vi "Write Center Point.vi"(10 "Center Point":dbl[unit], 11 "PressureServoActuator in":refnum<class "PressureServoActuator.lvclass">) -> (3 "PressureServoActuator out":refnum<class "PressureServoActuator.lvclass">)   [LabVIEW 2015, in "PressureServoActuator.lvclass"]
uses:
  PressureServoActuator.lvclass
  PressureServoActuator.lvclass/PressureServoActuator.ctl
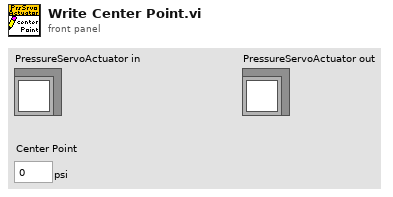
[diagram p1: front panel]
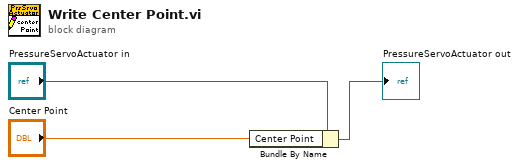
[diagram p0: block diagram]
diagram:
  n1 = Bundle By Name(cluster="PressureServoActuator in", "Center Point"="Center Point") -> (→"PressureServoActuator out":refnum<class "PressureServoActuator.lvclass">)
